vi "Sweep Level And Frequency.vi"(0 "VISA resource name":refnum<visa-resource-name>, 1 "Step/Number Of Points (F:Points)":bool, 2 "Sweep Definition (T:Start/Stop)":bool=TRUE, 3 "Sweep (0:Frequency [Hz])":u32(ring) items=["Frequency [Hz]", "DC Bias [V]", "Oscilator Level [V]", "Oscilator Level [dBm]", "Oscilator Level [dBV]"], 5 "Start/Center (10,00E-3)":dbl=10000.0 min=-40.0 max=40000000.0 format="%^.3e", 7 "Stop/Span (10,00E-3)":dbl=10000.0 min=-40.0 max=40000000.0 format="%^.3e", 9 "Step (10,00E-3)":dbl=10000.0 min=0.001 max=99999.0 format="%^.3e", 11 "error in (no error)":errorcluster, 12 "Number Of Points (100)":i32=100 min=2 max=401) -> (4 "VISA resource name out":refnum<visa-resource-name>, 15 "error out":errorcluster)   [LabVIEW 2011, in "Agilent 4194.lvlib"]
doc: "This function sets the sweep parameters."
uses:
  <instrlib>/Agilent 4194/Agilent 4194.lvlib
panel:
  # "Start/Stop"
  # "Center/Spen"
  # "Step"
  # "Points"
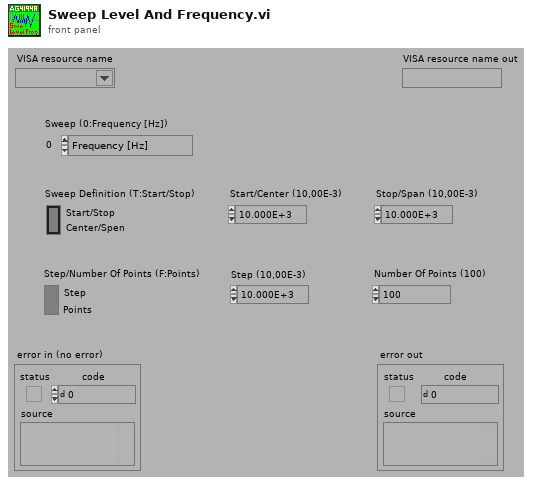
[diagram p1: front panel]
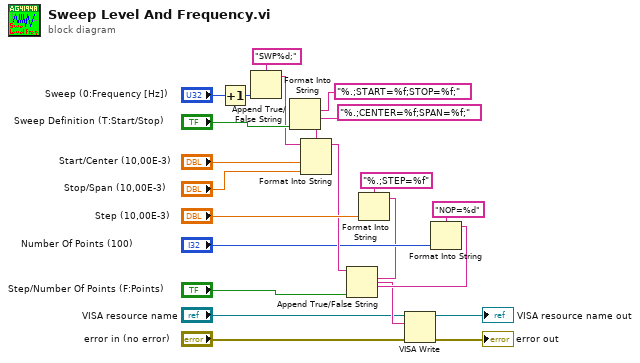
[diagram p0: block diagram]
diagram:
  n1 = Increment(x="Sweep (0:Frequency [Hz])") -> (x+1=w1:u32)
  n2 = Format Into String(format string="SWP%d;", w1) -> (resulting string=w15:string)  [unwired: 2 in, 1 out]
  n3 = Append True/False String(1:"Sweep Definition (T:Start/Stop)", 2:"%.;CENTER=%f;SPAN=%f;", 3:"%.;START=%f;STOP=%f;") -> (0:w16:string)  [unwired: 1 in]
  n4 = Format Into String(format string=w16, initial string=w15, "Start/Center (10,00E-3)", "Stop/Span (10,00E-3)") -> (resulting string=w12:string)  [unwired: 1 in, 1 out]
  n5 = Format Into String(format string="%.;STEP=%f", "Step (10,00E-3)") -> (resulting string=w8:string)  [unwired: 2 in, 1 out]
  n6 = Format Into String(format string="NOP=%d", "Number Of Points (100)") -> (resulting string=w7:string)  [unwired: 2 in, 1 out]
  n7 = Append True/False String(1:"Step/Number Of Points (F:Points)", 2:w7, 3:w8, 4:w12) -> (0:w6:string)
  n8 = VISA Write(VISA resource name="VISA resource name", write buffer=w6, error in (no error)="error in (no error)") -> (VISA resource name out=→"VISA resource name out":refnum<visa-resource-name>, error out=→"error out":errorcluster)  [unwired: 1 out]
